vi "Initialize Network.vi"() -> (0 "error out":errorcluster, 3 "UDP Network Connection out":refnum<k16>)   [LabVIEW 2015]
doc: "This is where we generally initialize network associated things. This includes all shared variables not referenced in the configuration file and a possible UDP connection which broadcasts the address of the controller.\n\nAs of 10 October 2016, the UDP functionality is not implemented but is sketched out."
uses:
  <vilib>/Utility/tcp.llb/UDP Multicast Write-Only Open.vi
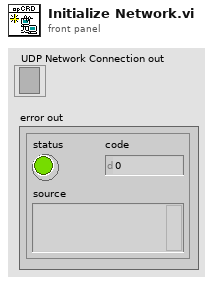
[diagram p1: front panel]
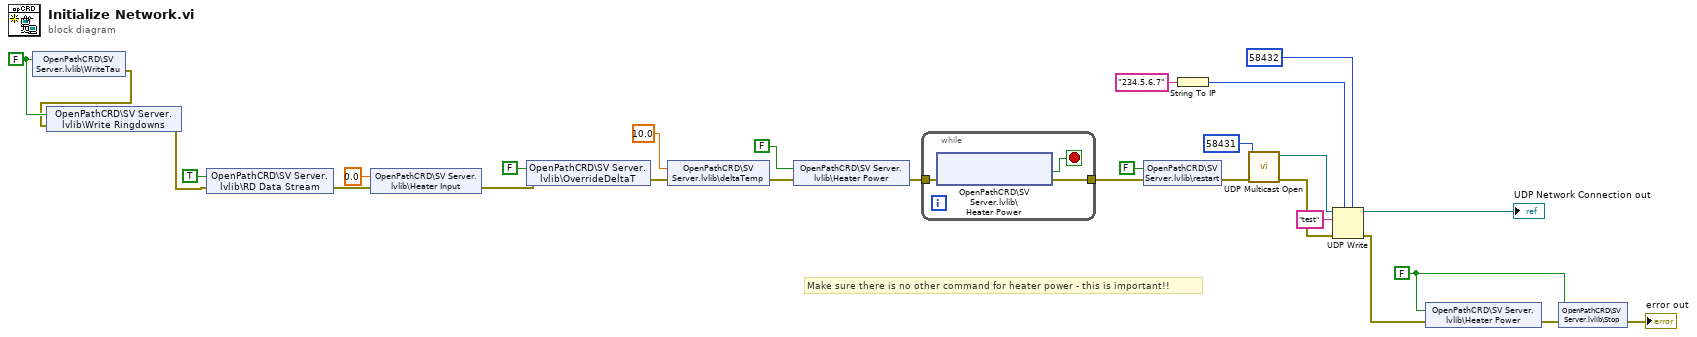
[diagram p0: block diagram]
diagram:
  w3 = FALSE ("WriteTau")
  w10 = FALSE ("Stop")
  # "Make sure there is no other command for heater power - this is important!!"
  n1 = shared-variable "OpenPathCRD\\SV Server.lvlib\\WriteTau"(w3) -> (error out=w2:errorcluster)  [unwired: 1 in]
  n2 = shared-variable "OpenPathCRD\\SV Server.lvlib\\Write Ringdowns"(w3, error in=w2) -> (error out=w1:errorcluster)
  n3 = shared-variable "OpenPathCRD\\SV Server.lvlib\\RD Data Stream"(TRUE ("RD Data Stream"), error in=w1) -> (error out=w5:errorcluster)
  n4 = shared-variable "OpenPathCRD\\SV Server.lvlib\\Heater Input"(0.0 ("Heater Input"), error in=w5) -> (error out=w4:errorcluster)
  n5 = shared-variable "OpenPathCRD\\SV Server.lvlib\\OverrideDeltaT"(FALSE ("OverrideDeltaT"), error in=w4) -> (error out=w28:errorcluster)
  n6 = shared-variable "OpenPathCRD\\SV Server.lvlib\\deltaTemp"(10.0 ("deltaTemp"), error in=w28) -> (error out=w25:errorcluster)
  n7 = shared-variable "OpenPathCRD\\SV Server.lvlib\\Heater Power"(FALSE ("Stop"), error in=w25) -> (error out=w23:errorcluster)
  n8 = while {
    tunnel: w23 -> [w30]
    tunnel: [w29] -> w24
    stop <- w31 stop-if-true
    n9 = shared-variable "OpenPathCRD\\SV Server.lvlib\\Heater Power"(error in=w30) -> (error out=w29:errorcluster, w31:bool)  [unwired: 1 in, 1 out]
  }
  n10 = shared-variable "OpenPathCRD\\SV Server.lvlib\\restart"(FALSE ("restart"), error in=w24) -> (error out=w21:errorcluster)
  n11 = String To IP(1:"234.5.6.7" ("name")) -> (0:w15:u32)
  n12 = call-poly <vilib>:"UDP Multicast Open.vi"("error in (no error)"=w21, "port"=u16 58431) -> ("error out"=w14:errorcluster, "connection ID"=w13:refnum<k16>)  [unwired: 8 in]
  n13 = UDP Write(address=w15, port or service name=u16 58432, connection ID=w13, data in="test", 8:w14) -> (error out=w17:errorcluster, 3:→"UDP Network Connection out":refnum<k16>)  [unwired: 1 in]
  n14 = shared-variable "OpenPathCRD\\SV Server.lvlib\\Heater Power"(w10, error in=w17) -> (error out=w9:errorcluster)
  n15 = shared-variable "OpenPathCRD\\SV Server.lvlib\\Stop"(w10, error in=w9) -> (error out=→"error out":errorcluster)
